vi "Mode Est Process Data.vi"(8 "error in (no error)":errorcluster, 9 "Damping Ratio History":dbl[][](array[numeric]), 10 "Mode Estimator Processing Settings":T3={"Low-Pass Filter Order"=5, "Downsampling Ratio"=10.0, "LPF Cut-off Frequency [Hz]"=2.5, "Sampling Frequency (Hz)"=50.0, "Parcel Length (Simulation)"=30000, "Detrend Cut-off Frequency (Hz)"=0.05, "AR Order"=25, "MA Order "=10, "Lower Frequency [Hz]"=0.08, "Upper Frequency [Hz]"=2.0, "Upper Damping [%]"=20.0, "Lower Damping [%]"=0.0, "Std Threshold"=1.35, "Length of Spectra [s]"=12.0, "Refresh Rate [s]"=0, "Number of critical modes"=1}, 11 "Waveform in":waveform(dbl)) -> (0 "error out":errorcluster, 1 "Display Data B":T2={"Damping ratio evolution"=[], "Estimated Complex Plane"={[], []}, "Critical Frequency [Hz]"=0.0, "Critical Damping [%]"=0.0, " Complex Poles"=[0.0+0.0i, 0.0+0.0i, 0.0+0.0i], "Damping Ratio [%]"=[0.0, 0.0, 0.0], " Frequency[Hz]"=[0.0, 0.0, 0.0], "Mean Damping [%]"=[0.0, 0.0, 0.0], "Pictures"=[bytes[260130], bytes[260130], bytes[260130]], "Std of Damping"=[0.0, 0.0, 0.0]} {"Frequency[Hz]" format="%.4f"; "Damping Ratio [%]" format="%.4f"; "Complex Poles" format="%.4f"}, 3 "Display Data A":T1={"Real-time data"={"t0"=timestamp(3467964116.0127993 s since 1904-01-01), "dt"=0.02, "Y"=array[30000 elements]}, "Preprocessed data"={"t0"=timestamp(3467964116.0127993 s since 1904-01-01), "dt"=0.2, "Y"=array[3000 elements]}, "ARMA Transfer Function"=bytes[0], "Spectrogram"=[refnum], "Spectrum"={"f0"=0.0, "df"=0.0048828125, "S(f)"=[]}, "Parcel Length (SDK or Simulation)"=30000})   [LabVIEW 2017]
uses:
  Mode Est Processing Settings.ctl
  Display Data B.ctl
  Display Data A.ctl
  <vilib>/Math Plots/3D Math Plots/3D Surface/3D Surface Datatype/3D Surface Datatype.lvclass
  <vilib>/Math Plots/3D Math Plots/3D Surface/3D Surface XCtrl/3D Surface.xctl
  Processing State.ctl
  <vilib>/Math Plots/3D Math Plots/3D Plot/3D Plot Datatype/3D Plot Datatype.lvclass
  <vilib>/addons/Wavelet Analysis/application.llb/WA Detrend (Waveform).vi
  Program Files (x86)/National Instruments/LabVIEW 2017/vi.lib/addons/System Identification/Data Preprocess.llb/SI Lowpass Filter (SISO Waveform).vi
  <vilib>/addons/Time Series Analysis/Modeling and Prediction.llb/TSA ARMA Modeling (Waveform).vi
  <vilib>/addons/Control Design/_Model Construction/Model Creation.llb/Model Creation SubVI/cd_Create Transfer Function Model.vi
  <vilib>/addons/Control Design/_Utility/Model Viewer.llb/Model Viewer SubVI/cd_Draw Transfer Function Equation (TF).vi
  <vilib>/addons/Control Design/_Model Conversions/Continuous and Discrete.llb/Continuous and Discrete SubVI/cd_Convert Discrete to Continuous (TF).vi
  <vilib>/addons/Control Design/_Model Conversions/Model Type.llb/Model Conversion SubVI/cd_Convert Transfer Function to State-Space Model.vi
  <vilib>/addons/Control Design/_Dynamic Analysis/Dynamic Analysis.llb/Dynamic Analysis subVI/cd_Damping Ratio and Natural Frequency (State-Space).vi
  <vilib>/imath/engines/lvmath2/RunTimeEngine/Managers/WorkSpace/UID Generator.vi
  <vilib>/imath/engines/lvmath2/RunTimeEngine/BuiltInFunctions/sort/NIMS_[2o]_sort(RRowV,I32,Str).vi
  <instcachedir>/0/NIMS_[2o]_sort(RRowV,I32,Str)_E84E23B068DF4763991B1E74560868DE.lvgen/NIMS_[2o]_sort(RRowV,I32,Str)_E84E23B068DF4763991B1E74560868DE_000.vi
  <vilib>/imathl/engines/lvmath/Functions/Error Handling/Create Error.vi
  <vilib>/imath/engines/lvmath2/RunTimeEngine/IndexRead/NIMS V(V).vi
  <instcachedir>/0/NIMS V(V)_298D9CB7BFEB42B8BC8D9C3C28AE8C70.lvgen/NIMS V(V)_298D9CB7BFEB42B8BC8D9C3C28AE8C70_000.vi
  <instcachedir>/0/NIMS V(V)_298D9CB7BFEB42B8BC8D9C3C28AE8C70.lvgen/NIMS V(V)_298D9CB7BFEB42B8BC8D9C3C28AE8C70_001.vi
  <vilib>/imath/engines/lvmath2/RunTimeEngine/BitwiseOperatorToken/NIMS_Bitwise_Operator_And.vi
  <instcachedir>/0/NIMS_Bitwise_Operator_And_BF79565AECDF4B89921EA9614C6BB008.lvgen/NIMS_Bitwise_Operator_And_BF79565AECDF4B89921EA9614C6BB008_001.vi
  <vilib>/imath/engines/lvmath2/RunTimeEngine/BuiltInFunctions/imag/NIMS_imag(Complex).vi
  <instcachedir>/0/NIMS_imag(Complex)_3180D40D00C843A49C2B33397F857BF3.lvgen/NIMS_imag(Complex)_3180D40D00C843A49C2B33397F857BF3_002.vi
  <vilib>/imath/engines/lvmath2/RunTimeEngine/BuiltInFunctions/findnz/NIMS_[1o]_findnz(GRowV).vi
  <instcachedir>/0/NIMS_[1o]_findnz(GRowV)_4566141FE5BA40B7B10E18ED0AB78B2D.lvgen/NIMS_[1o]_findnz(GRowV)_4566141FE5BA40B7B10E18ED0AB78B2D_000.vi
  <vilib>/imath/engines/lvmath2/RunTimeEngine/RunTimeType/NIMS_RunTimeType_From StrictType (excl LVString).vi
  <instcachedir>/0/NIMS_RunTimeType_From StrictType (excl LVString)_DC56D72BB6B948F98D63F1A957D87C42.lvgen/NIMS_RunTimeType_From StrictType (excl LVString)_DC56D72BB6B948F98D63F1A957D87C42_000.vi
  <vilib>/imath/engines/lvmath2/RunTimeEngine/ErrorHandling/NIMS_Create Error From Enums.vi
  <vilib>/imath/engines/lvmath2/RunTimeEngine/LocalVariableDefStatement/MC_LocalVariableDefStatement_Display.vi
  <vilib>/imath/engines/lvmath2/RunTimeEngine/Managers/SymbolTable/Clear UID.vi
  <vilib>/imath/engines/lvmath2/RunTimeEngine/NodeEndStatement/NIMS_NodeEndStatement_Output.vi
  <instcachedir>/0/NIMS_NodeEndStatement_Output_53EC0D466D134D7ABD903AC30B43404B.lvgen/NIMS_NodeEndStatement_Output_53EC0D466D134D7ABD903AC30B43404B_005.vi
  <instcachedir>/0/NIMS_NodeEndStatement_Output_53EC0D466D134D7ABD903AC30B43404B.lvgen/NIMS_NodeEndStatement_Output_53EC0D466D134D7ABD903AC30B43404B_000.vi
  <vilib>/imath/engines/lvmath2/RunTimeEngine/ErrorHandling/NIMS_Finalize Error.vi
  <vilib>/addons/Time Series Analysis/Correlation and Spectral Analysis.llb/TSA ARMA Spectrum (Waveform).vi
  <vilib>/imath/engines/lvmath2/RunTimeEngine/RangeToken/NIMS_Range.vi
  <instcachedir>/0/NIMS_Range_8C005833F4504FD4A29AA23D6150121A.lvgen/NIMS_Range_8C005833F4504FD4A29AA23D6150121A_000.vi
  <vilib>/imath/engines/lvmath2/RunTimeSupport/NIMS_Error if Not Equal.vi
  <instcachedir>/0/NIMS_Error if Not Equal_E5646C1EFB50404BB0542B8CFB81CE27.lvgen/NIMS_Error if Not Equal_E5646C1EFB50404BB0542B8CFB81CE27_001.vi
  <instcachedir>/0/NIMS_Error if Not Equal_E5646C1EFB50404BB0542B8CFB81CE27.lvgen/NIMS_Error if Not Equal_E5646C1EFB50404BB0542B8CFB81CE27_000.vi
  <vilib>/imath/engines/lvmath2/RunTimeEngine/IndexRead/NIMS V($).vi
  <instcachedir>/0/NIMS V($)_C593F32C7F6B43C7B1793952E292524F.lvgen/NIMS V($)_C593F32C7F6B43C7B1793952E292524F_001.vi
  <vilib>/imath/engines/lvmath2/RunTimeEngine/IndexReplace/NIMS M(S,$)=V.vi
  <instcachedir>/0/NIMS M(S,$)=V_552265ADF67C4F4FB07E91CD22492551.lvgen/NIMS M(S,$)=V_552265ADF67C4F4FB07E91CD22492551_000.vi
  <vilib>/imath/engines/lvmath2/RunTimeEngine/IndexReplace/NIMS V(S)=S.vi
  <instcachedir>/0/NIMS V(S)=S_EDDEB2B900FD4B108B325BCE58B17C3D.lvgen/NIMS V(S)=S_EDDEB2B900FD4B108B325BCE58B17C3D_000.vi
  <vilib>/imath/engines/lvmath2/RunTimeEngine/IndexReplace/NIMS V(V)=V.vi
  <instcachedir>/0/NIMS V(V)=V_ACB9F458E2974419B362D656D10048D7.lvgen/NIMS V(V)=V_ACB9F458E2974419B362D656D10048D7_000.vi
  <vilib>/imath/engines/lvmath2/RunTimeEngine/IndexRead/NIMS M(V,$).vi
  <instcachedir>/0/NIMS M(V,$)_21A5155762F74C04AE4EA67BEE0D3EF5.lvgen/NIMS M(V,$)_21A5155762F74C04AE4EA67BEE0D3EF5_004.vi
  <instcachedir>/0/NIMS_NodeEndStatement_Output_53EC0D466D134D7ABD903AC30B43404B.lvgen/NIMS_NodeEndStatement_Output_53EC0D466D134D7ABD903AC30B43404B_009.vi
  <instcachedir>/0/NIMS_NodeEndStatement_Output_53EC0D466D134D7ABD903AC30B43404B.lvgen/NIMS_NodeEndStatement_Output_53EC0D466D134D7ABD903AC30B43404B_002.vi
  <instcachedir>/0/NIMS_NodeEndStatement_Output_53EC0D466D134D7ABD903AC30B43404B.lvgen/NIMS_NodeEndStatement_Output_53EC0D466D134D7ABD903AC30B43404B_001.vi
  <vilib>/Math Plots/3D Math Plots/3D Surface/3D Surface Datatype/Public/Plot Helper (Vector).vi
  <vilib>/addons/Control Design/_Model Construction/Data Typedefs.llb/CD DtoC Conversion Method.ctl
  Program Files (x86)/National Instruments/LabVIEW 2017/vi.lib/addons/System Identification/NI_SysID.lvlib
  <vilib>/addons/_Advanced Signal Processing/NI_AdvSigProcWA.lvlib
  <vilib>/addons/_Advanced Signal Processing/NI_AdvSigProcTSA.lvlib
  <vilib>/addons/Control Design/_Model Construction/NI_LinSys_Model Creation.lvlib
  <vilib>/addons/Control Design/_Model Conversions/NI_CD_Continuous and Discrete.lvlib
  <vilib>/addons/Control Design/_Model Construction/NI_LinSys_Data Typedefs.lvlib
  <vilib>/addons/Control Design/_Dynamic Analysis/NI_CD_Dynamic Analysis.lvlib
  <vilib>/Analysis/NI_AALBase.lvlib
  <vilib>/addons/Control Design/_Model Conversions/NI_CD_Model Type.lvlib
  <vilib>/imath/engines/lvmath2/RunTimeEngine/Managers/SymbolTable/NIMS_WorkSpace.lvlib
  <vilib>/addons/Control Design/_Utility/NI_CD_Model Viewer.lvlib
panel:
  # "MA\n_______\n\n   AR"
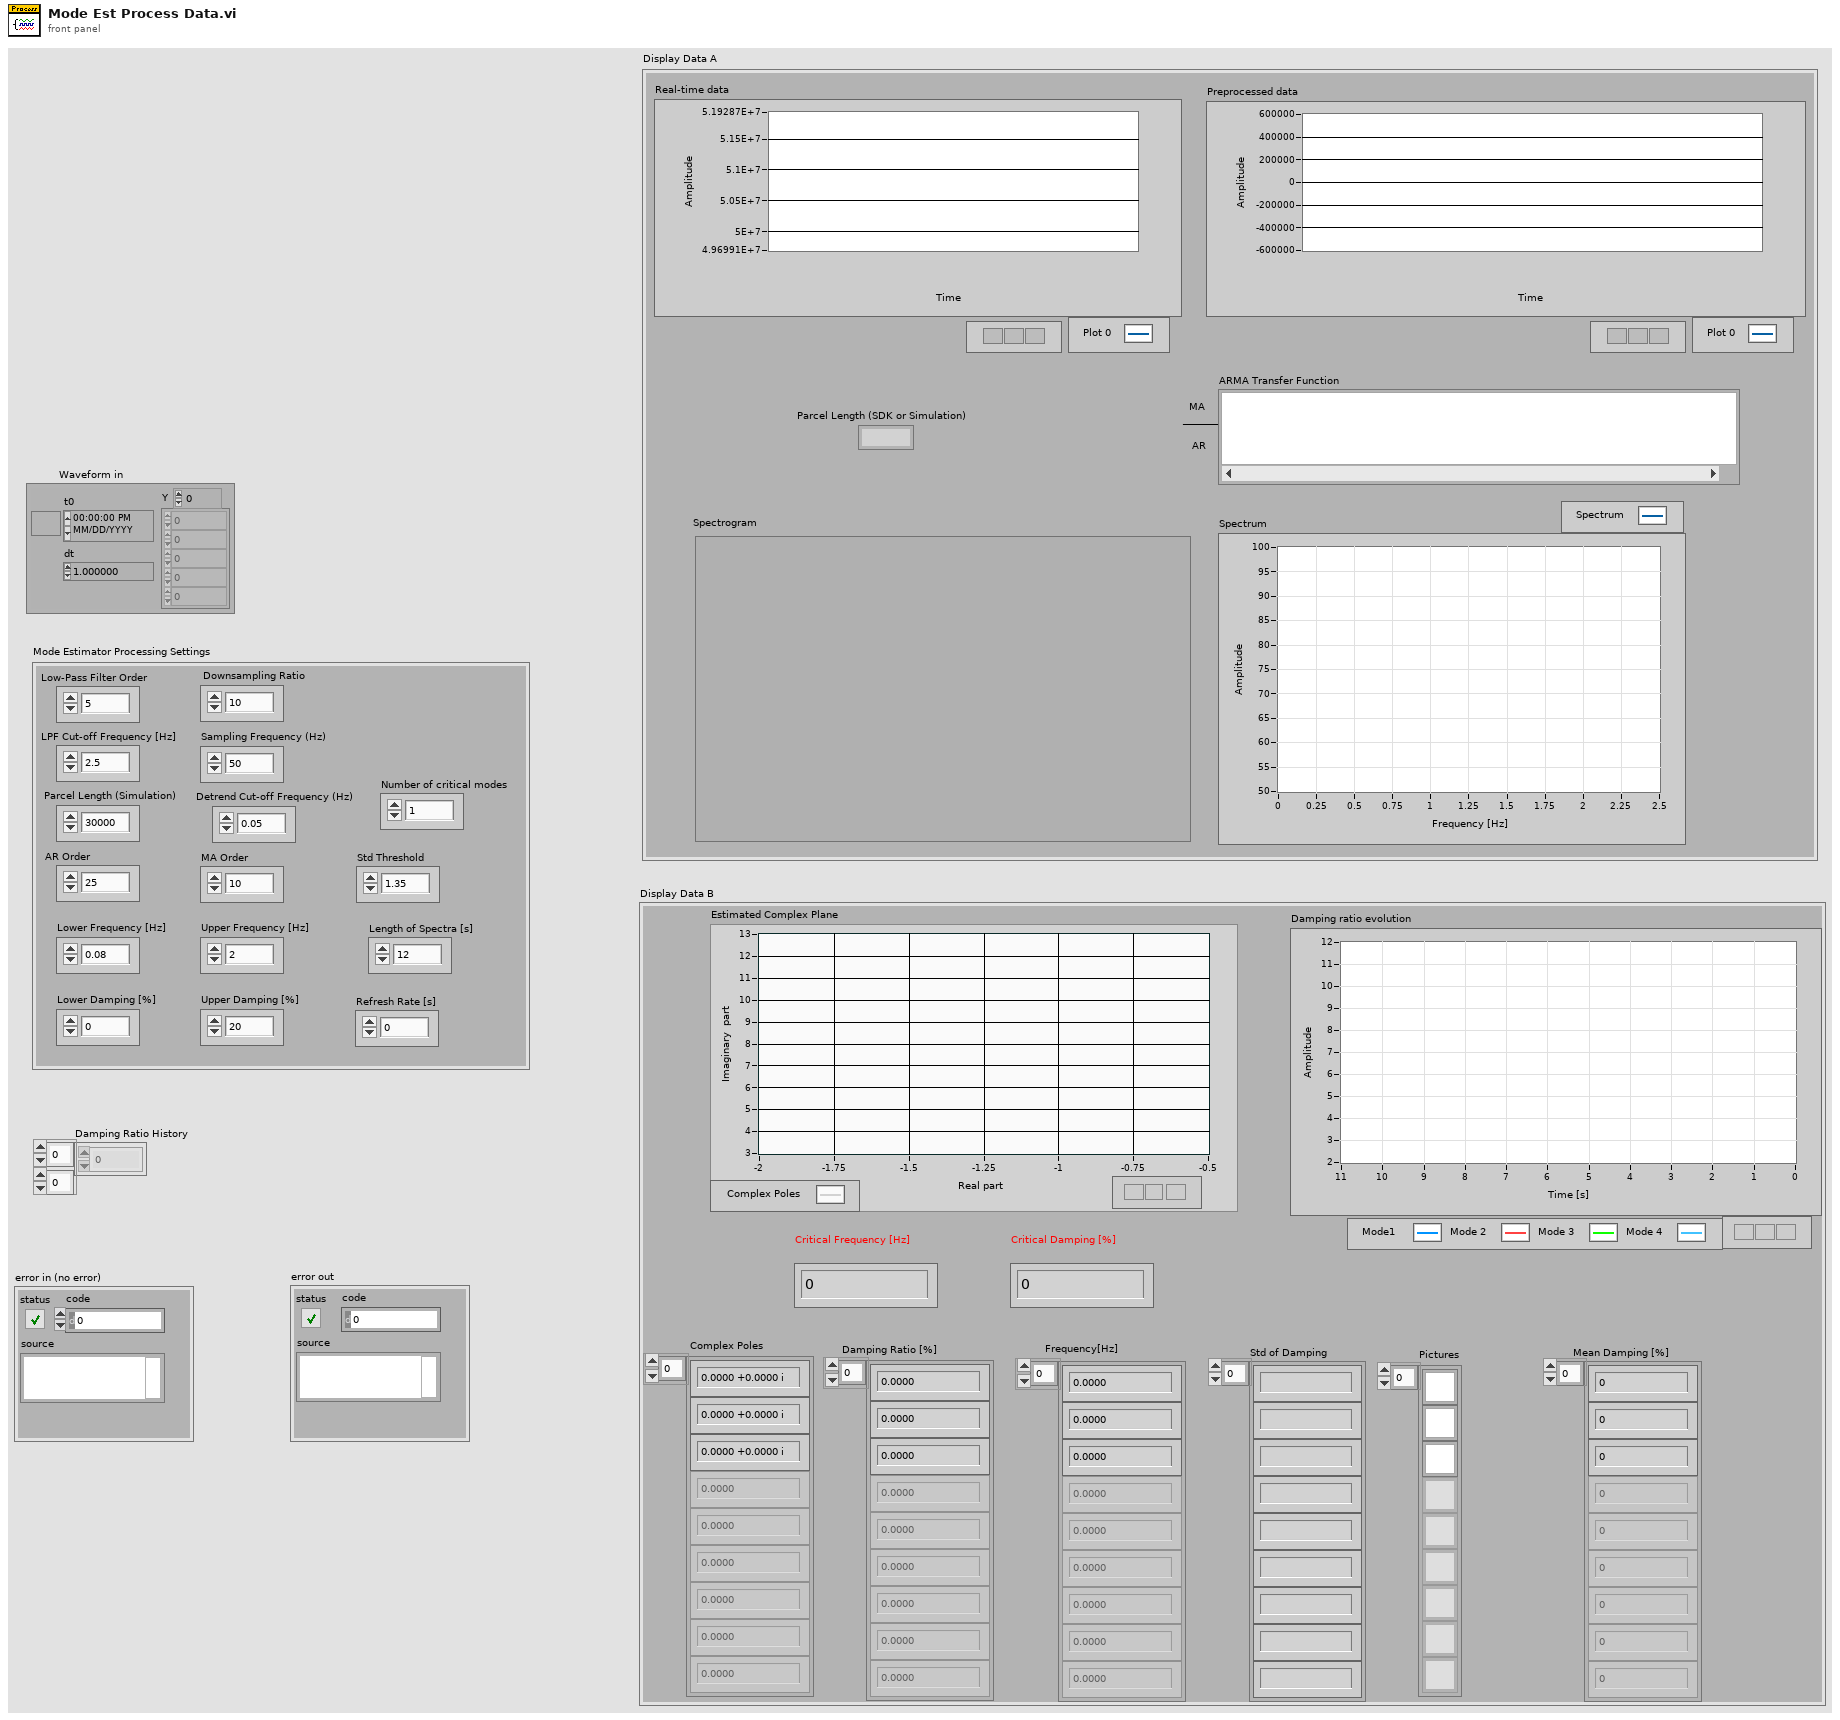
[diagram p1: front panel]
types:
  T1 = typedef "Display Data A.ctl" = cluster{"Real-time data":waveform(dbl), "Preprocessed data":waveform(dbl), "ARMA Transfer Function":picture, "Spectrogram":refnum<class "3D Plot Datatype.lvclass">[], "Spectrum":cluster{"f0":dbl, "df":dbl, "S(f)":dbl[]}, "Parcel Length (SDK or Simulation)":i32}
  T2 = typedef "Display Data B.ctl" = cluster{"Damping ratio evolution":dbl[][], "Estimated Complex Plane":cluster{dbl[], dbl[]}, "Critical Frequency [Hz]":dbl, "Critical Damping [%]":dbl, " Complex Poles":cdb[], "Damping Ratio [%]":dbl[], " Frequency[Hz]":dbl[], "Mean Damping [%]":dbl[], "Pictures":picture[], "Std of Damping":dbl[]}
  T3 = typedef "Mode Est Processing Settings.ctl" = cluster{"Low-Pass Filter Order":i32, "Downsampling Ratio":dbl, "LPF Cut-off Frequency [Hz]":dbl, "Sampling Frequency (Hz)":dbl, "Parcel Length (Simulation)":i32, "Detrend Cut-off Frequency (Hz)":dbl, "AR Order":i32, "MA Order ":i32, "Lower Frequency [Hz]":dbl, "Upper Frequency [Hz]":dbl, "Upper Damping [%]":dbl, "Lower Damping [%]":dbl, "Std Threshold":dbl, "Length of Spectra [s]":dbl, "Refresh Rate [s]":i32, "Number of critical modes":i32}
  T4 = typedef "Processing State.ctl" = enum16{"Preprocessing", "Compute AR Coeff", "Get Spectrum"}
  T5 = cluster{"Damping ratio evolution":dbl[][], "Estimated Complex Plane":cluster{dbl[], dbl[]}, "Critical Frequency [Hz]":dbl, "Critical Damping [%]":dbl, " Complex Poles":cdb[], "Damping Ratio [%]":dbl[], " Frequency[Hz]":dbl[], "Mean Damping [%]":dbl[], "Pictures":picture[], "Std of Damping":dbl[]}
  T6 = typedef "NI_LinSys_Data Typedefs.lvlib/CD DtoC Conversion Method.ctl" = u16
  T7 = typedef "NI_LinSys_Model Typedefs.lvlib/CD Transfer Function Model (MIMO).ctl" = cluster{"properties":T8, "transfer function(s)":T9[][]}
  T8 = typedef "NI_LinSys_Model Typedefs.lvlib/CD General Elements.ctl" = cluster{"Model name":string, "Input names":string[], "Output names":string[], "Input Delays":dbl[], "Output Delays":dbl[], "Sampling Time":dbl, "Notes":string}
  T9 = typedef "NI_LinSys_Model Typedefs.lvlib/CD Transfer Function Model (SISO).ctl" = cluster{"Numerator":dbl[], "Denominator":dbl[], "delay":dbl}
  T10 = typedef "NI_LinSys_Model Typedefs.lvlib/CD State Space Model (MIMO).ctl" = cluster{"properties":T8, "A":dbl[][], "B":dbl[][], "C":dbl[][], "D":dbl[][], "StateNames":string[], "Transport Delay":dbl[][]}
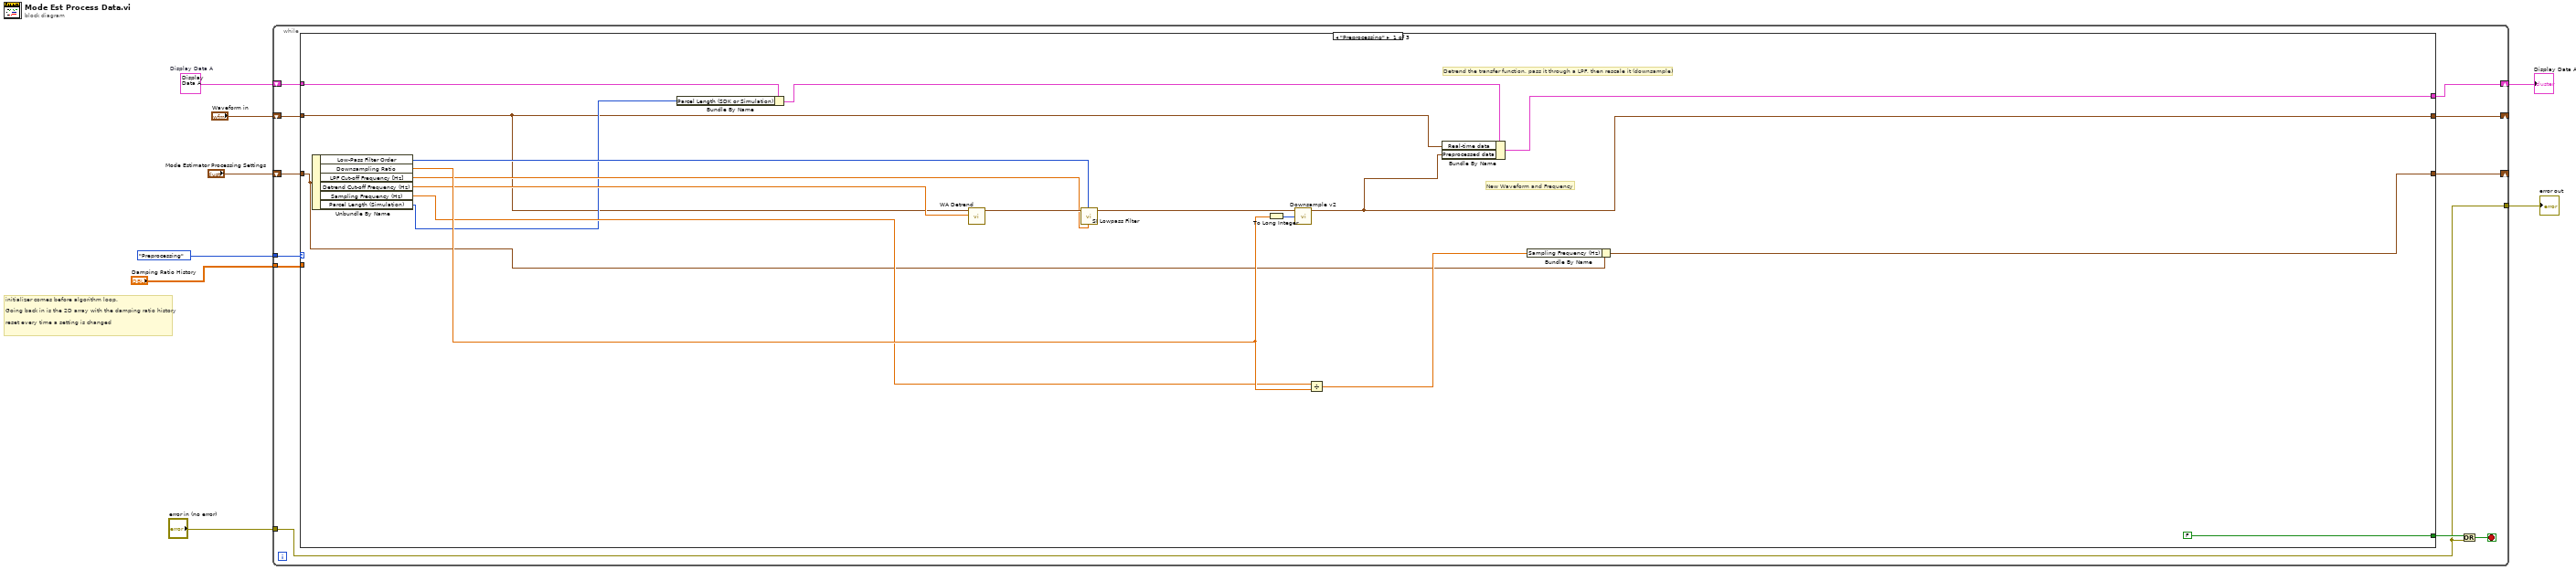
[diagram p0: block diagram]
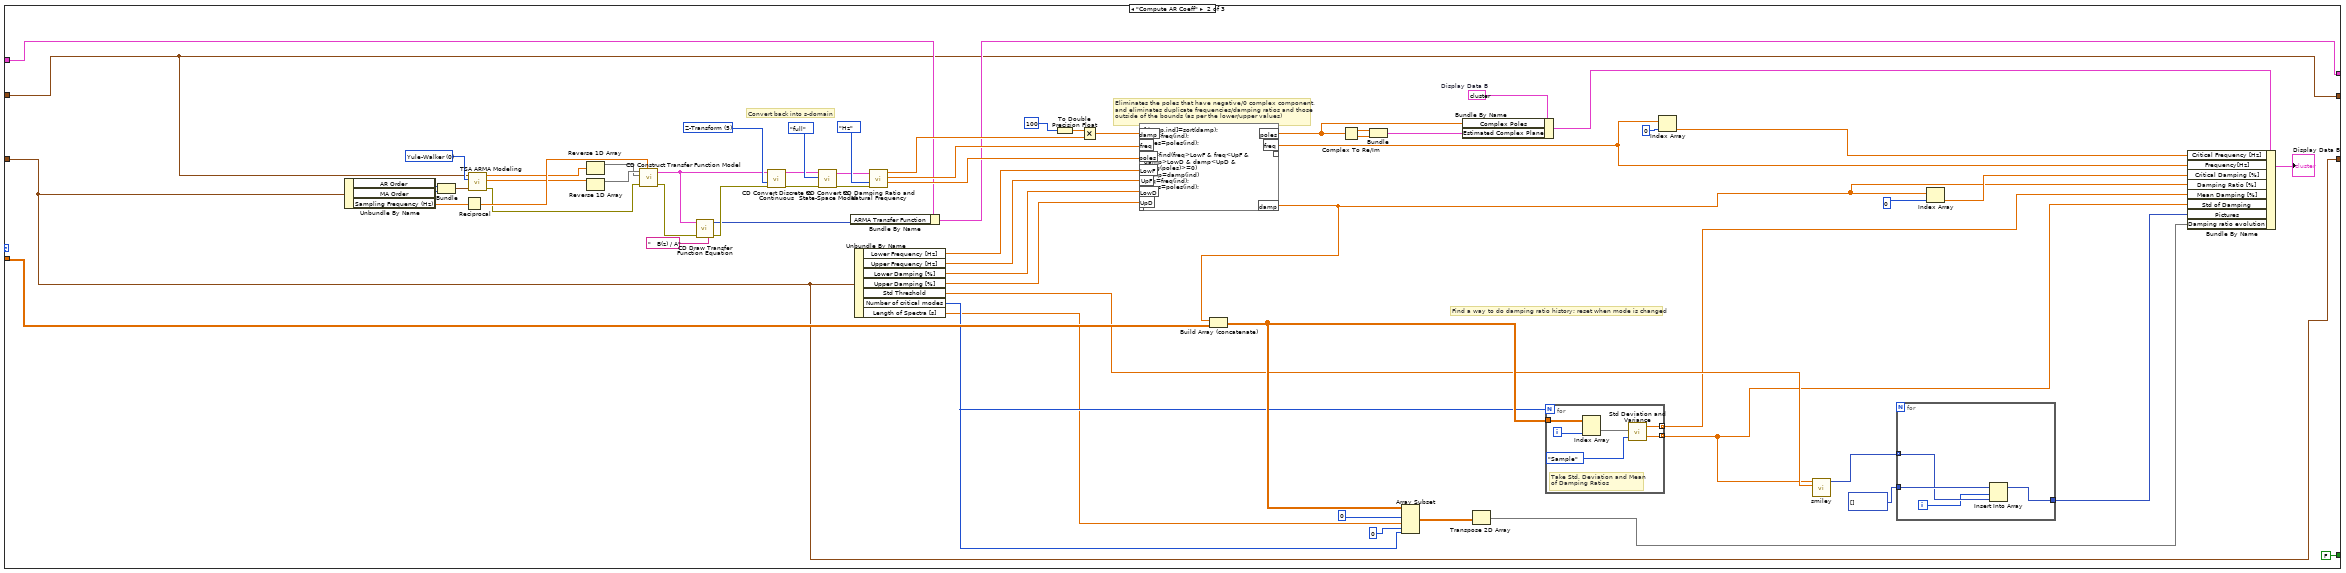
[diagram p2: hidden frame]
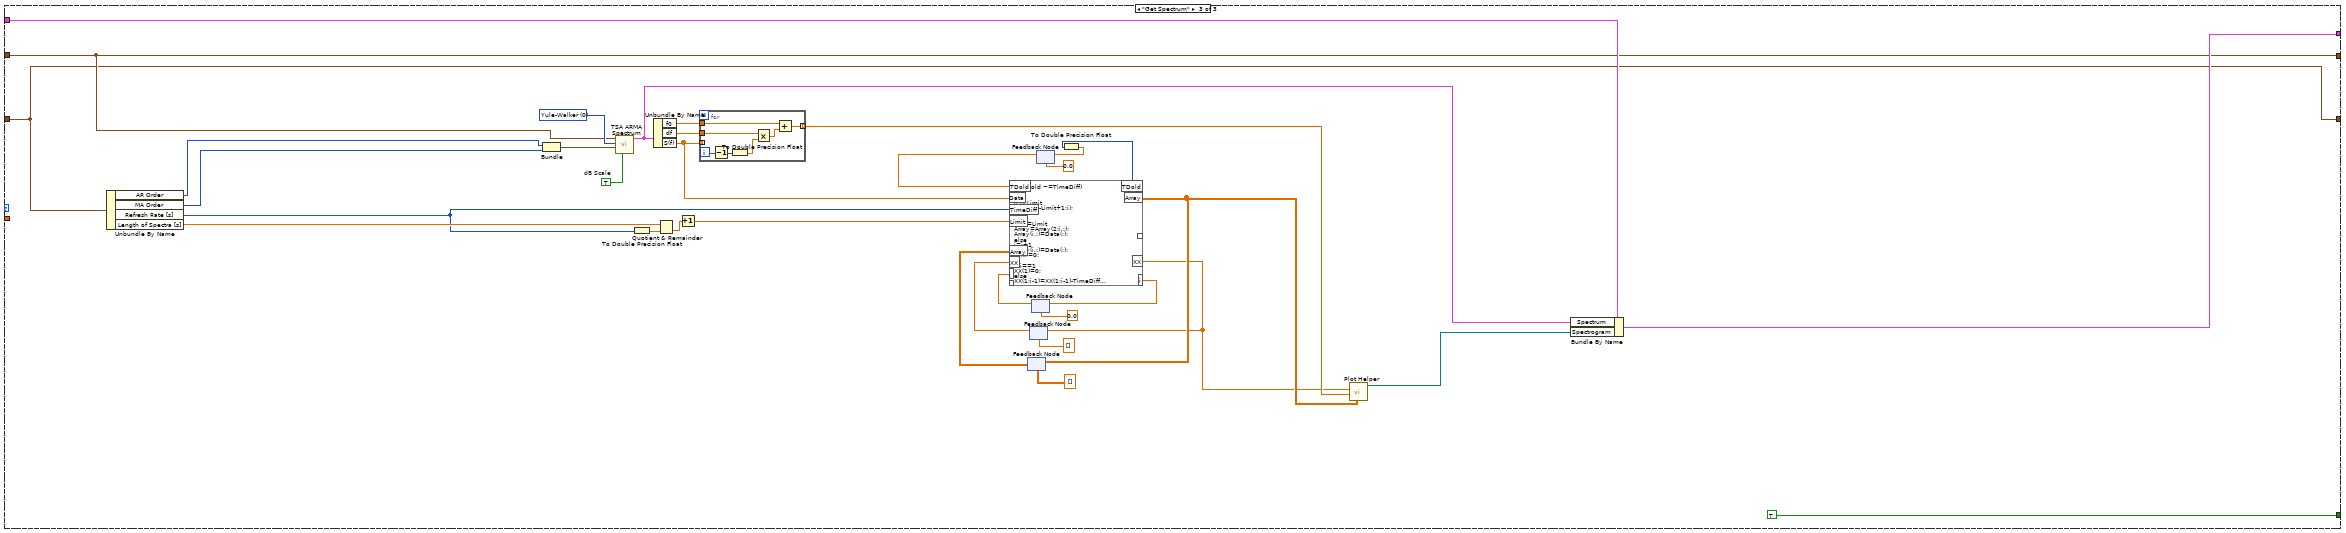
[diagram p3: hidden frame]
diagram:
  w4 = T1 {"Real-time data"={"t0"=timestamp(3467964116.0127993 s since 1904-01-01), "dt"=0.02, "Y"=array[30000 elements]}, "Preprocessed data"={"t0"=timestamp(3467964116.0127993 s since 1904-01-01), "dt"=0.2, "Y"=array[3000 elements]}, "ARMA Transfer Function"=bytes[0], "Spectrogram"=[refnum], "Spectrum"={"f0"=0.0, "df"=0.0048828125, "S(f)"=[]}, "Parcel Length (SDK or Simulation)"=30000}  # Display Data A
  # "initializer comes before algorithm loop.\n\nGoing back in is the 2D array with the damping ratio history\n\nreset every time a setting is changed"
  n1 = while {
    tunnel: "Damping Ratio History" -> [w19]
    tunnel: Processing_State."Preprocessing" ("Enum") -> [w17]
    shift-right: [w16] -> _
    shift-left: "Waveform in" -> [w10]
    shift-right: [w15] -> w5
    shift-left: w4 -> [w14]
    tunnel: "error in (no error)" -> [w11]
    tunnel: [w11] -> w2
    shift-right: [w9] -> _
    shift-left: "Mode Estimator Processing Settings" -> [w18]
    stop <- w12 stop-if-true
    n2 = case shown="\"Preprocessing\"" w17 {
      tunnel: w10 -> [w26 w39 w330]
      tunnel: [w21 w39 w330] -> w16
      tunnel: w19 -> [_ w96 _]
      tunnel: w18 -> [w23 w38 w329]
      tunnel: [FALSE FALSE TRUE] -> w13
      tunnel: w14 -> [w30 w41 w334]
      tunnel: [w31 w40 w333] -> w15
      tunnel: [w24 w38 w329] -> w9
      frame "Preprocessing" {
        # "New Waveform and Frequency"
        # "Detrend the transfer function, pass it through a LPF, then rescale it (downsample)"
        n3 = Unbundle By Name(w23) -> ("Low-Pass Filter Order"=w36:i32, "Downsampling Ratio"=w35:dbl, "LPF Cut-off Frequency [Hz]"=w34:dbl, "Detrend Cut-off Frequency (Hz)"=w33:dbl, "Sampling Frequency (Hz)"=w28:dbl, "Parcel Length (Simulation)"=w27:i32)
        n4 = Bundle By Name(cluster=w30, "Parcel Length (SDK or Simulation)"=w27) -> (w29:T1)
        n5 = call-poly <vilib>:"WA Detrend.vi"("threshold frequency"=w33, "signal"=w26) -> ("detrended signal"=w37:waveform(dbl))  [unwired: 7 in, 2 out]
        n6 = call-poly "SI Lowpass Filter.vi"("cutoff frequency"=w34, "order"=w36, "stimulus signal in"=w37) -> ("stimulus signal out"=w22:waveform(dbl))  [unwired: 6 in, 2 out]
        n7 = To Long Integer(number=w35) -> (32bit integer=w20:i32)
        n8 = call "Downsample v2.vi"("Divide by"=w20, "Waveform in"=w22) -> ("Waveform out"=w21:waveform(dbl))  [unwired: 9 in]
        n9 = Divide(x=w28, y=w35) -> (x/y=w25:dbl)
        n10 = Bundle By Name(cluster=w29, "Real-time data"=w26, "Preprocessed data"=w21) -> (w31:T1)
        n11 = Bundle By Name(cluster=w23, "Sampling Frequency (Hz)"=w25) -> (w24:T3)
      }
      frame "Compute AR Coeff" {
        w45 = T5 {"Damping ratio evolution"=[], "Estimated Complex Plane"={[], []}, "Critical Frequency [Hz]"=0.0, "Critical Damping [%]"=0.0, " Complex Poles"=[0.0+0.0i, 0.0+0.0i, 0.0+0.0i], "Damping Ratio [%]"=[0.0, 0.0, 0.0], " Frequency[Hz]"=[0.0, 0.0, 0.0], "Mean Damping [%]"=[0.0, 0.0, 0.0], "Pictures"=[bytes[260130], bytes[260130], bytes[260130]], "Std of Damping"=[0.0, 0.0, 0.0]}  # Display Data B
        w101 = T6 5 items=["Zero-Order-Hold", "Tustin (Bilinear)", "Prewarp", "Forward", "Backward", "Z-Transform"] ("Method")
        w102 = u16 0 items=["Yule-Walker", "High order AR", "Polynomial"] ("method")
        # "Find a way to do damping ratio history; reset when mode is changed"
        # "Convert back into s-domain"
        # "Eliminates the poles that have negative/0 complex component,\nand eliminates duplicate frequencies/damping ratios and those \noutside of the bounds (as per the lower/upper values)"
        n12 = Unbundle By Name(w38) -> ("AR Order"=w100:i32, "MA Order"=w76:i32, "Sampling Frequency (Hz)"=w74:dbl)
        n13 = Bundle("AR Order"=w100, "MA Order"=w76) -> (w99:cluster{"AR Order":i32, "MA Order ":i32})  [unwired: 1 in]
        n14 = Reciprocal(x=w74) -> (1/x=w75:dbl)
        n15 = call-poly <vilib>:"TSA ARMA Modeling.vi"("ARMA order"=w99, "method"=w102, "Xt"=w39) -> ("error out"=w66:errorcluster, "MA coefficients"=w71:dbl[], "AR coefficients"=w72:dbl[])  [unwired: 5 in, 1 out]
        n16 = Reverse 1D Array(array=w72) -> (reversed array=w88:dbl[])
        n17 = Reverse 1D Array(array=w71) -> (reversed array=w89:dbl[])
        n18 = call-poly <vilib>:"CD Construct Transfer Function Model.vi"("Sampling Time (s)"=w75, "error in (no error)"=w66, "Denominator"=w88, "Numerator"=w89) -> ("error out"=w68:errorcluster, "Transfer Function Model"=w70:T7)  [unwired: 6 in]
        n19 = call-poly <vilib>:"CD Draw Transfer Function Equation.vi"("Function Name (empty)"="   B(z) / A", "error in (no error)"=w68, "Transfer Function Model"=w70) -> ("error out"=w67:errorcluster, "Equation"=w42:picture)  [unwired: 6 in, 1 out]
        n20 = call-poly <vilib>:"CD Convert Discrete to Continuous.vi"("error in (no error)"=w67, "Method"=w101, "Discrete Transfer Function Model"=w70) -> ("error out"=w83:errorcluster, "Continuous Transfer Function Model"=w80:T7)  [unwired: 7 in]
        n21 = call-poly <vilib>:"CD Convert to State-Space Model.vi"("error in (no error)"=w83, "Realization Type"=enum16{"minimum", "full"}."full", "Transfer Function Model"=w80) -> ("error out"=w79:errorcluster, "State-Space Model"=w81:T10)  [unwired: 7 in]
        n22 = Bundle By Name(cluster=w41, "ARMA Transfer Function"=w42) -> (w40:T1)
        n23 = Unbundle By Name(w38) -> ("Lower Frequency [Hz]"=w62:dbl, "Upper Frequency [Hz]"=w63:dbl, "Lower Damping [%]"=w64:dbl, "Upper Damping [%]"=w65:dbl, "Std Threshold"=w59:dbl, "Number of critical modes"=w58:i32, "Length of Spectra [s]"=w57:dbl)
        n24 = call-poly <vilib>:"CD Damping Ratio and Natural Frequency.vi"("error in (no error)"=w79, "Frequency Unit"=enum16{"Hz", "rad/s"}."Hz", "State-Space Model"=w81) -> ("Poles"=w90:cdb[], "Natural Frequencies"=w84:dbl[], "Damping Ratios"=w93:dbl[])  [unwired: 5 in, 1 out]
        n25 = To Double Precision Float(number=100 ("Numeric")) -> (double precision float=w78:dbl)
        n26 = Multiply(x=w78, y=w93) -> (x*y=w92:dbl[])
        n27 = mathscript code="[damp,ind]=sort(damp);\nfreq=freq(ind);\npoles=poles(ind);\n\nind=find(freq>LowF & freq<UpF & damp>LowD & damp<UpD &  imag(poles)>=0)\ndamp=damp(ind)\nfreq=freq(ind);\npoles=poles(ind);"("damp"=w92, "freq"=w84, "poles"=w90, "LowF"=w62, "UpF"=w63, "LowD"=w64, "UpD"=w65) -> ("poles"=w52:cdb[], "freq"=w50:dbl[], "damp"=w49:dbl[])  [unwired: 1 in, 1 out]
        n28 = Build Array (concatenate) "Build Array"(w49, w96) -> (w61:dbl[][])
        n29 = Complex To Re/Im(x + iy=w52) -> (x=w98:dbl[], y=w97:dbl[])
        n30 = Bundle(w98, w97) -> (w56:cluster{dbl[], dbl[]})  [unwired: 1 in]
        n31 = Array Subset "Array Subset"(array=w61, index (row)=0 ("index"), length (row)=w57, index (col)=0 ("index"), length (col)=w58) -> (w73:dbl[][])
        n32 = Bundle By Name(cluster=w45, "Complex Poles"=w52, "Estimated Complex Plane"=w56) -> (w54:T5)
        n33 = Transpose 2D Array(2D array=w73) -> (transposed array=w48:dbl[][])
        n34 = for {
          N: w58 -> [_]
          tunnel: w61 -> [w111]
          tunnel: [w109] -> w47 mode=indexing
          tunnel: [w108] -> w43 mode=indexing
          i -> [w107]
          # "Take Std. Deviation and Mean\nof Damping Ratios"
          n35 = Index Array "Index Array"(array=w111, index (col)=w107) -> (element=w110:dbl[])  [unwired: 1 in]
          n36 = call <vilib>:"Std Deviation and Variance.vi"("X"=w110, "Weighting (Sample)"=enum16{"Sample", "Population"}."Sample") -> ("mean"=w109:dbl, "standard deviation"=w108:dbl)  [unwired: 1 out]
        }
        n37 = Index Array(array=w50, index=0) -> (element=w55:dbl)
        n38 = call "smiley.vi"("std threshold"=w59, "damp"=w43) -> ("Array"=w91:picture[])  [unwired: 9 in]
        n39 = for {
          tunnel: w91 -> [w105] mode=indexing
          tunnel: picture[] [] -> [w106]
          tunnel: [w103] -> w44
          i -> [w104]
          n40 = Insert Into Array(array=w106, index=w104, new element=w105) -> (w103:picture[])
        }
        n41 = Index Array(array=w49, index=0 ("length")) -> (element=w51:dbl)
        n42 = Bundle By Name(cluster=w54, "Critical Frequency [Hz]"=w55, "Frequency[Hz]"=w50, "Critical Damping [%]"=w51, "Damping Ratio [%]"=w49, "Mean Damping [%]"=w47, "Std of Damping"=w43, "Pictures"=w44, "Damping ratio evolution"=w48) -> (→"Display Data B":T5)
      }
      frame "Get Spectrum" {
        w355 = TRUE  # dB Scale
        w352 = u16 0 items=["Yule-Walker", "High order AR", "Polynomial"] ("method")
        n43 = Unbundle By Name(w329) -> ("AR Order"=w332:i32, "MA Order"=w331:i32, "Refresh Rate [s]"=w337:i32, "Length of Spectra [s]"=w338:dbl)
        n44 = Bundle("AR Order"=w332, "MA Order"=w331) -> (w362:cluster{"AR Order":i32, "MA Order ":i32})  [unwired: 1 in]
        n45 = call-poly <vilib>:"TSA ARMA Spectrum.vi"("dB on? (T)"=w355, "ARMA order"=w362, "method"=w352, "Xt"=w330) -> ("PSD"=w336:cluster{"f0":dbl, "df":dbl, "S(f)":dbl[]})  [unwired: 5 in, 2 out]
        n46 = To Double Precision Float(number=w337) -> (double precision float=w344:dbl)
        n47 = Unbundle By Name(w336) -> ("f0"=w360:dbl, "df"=w359:dbl, "S(f)"=w356:dbl[])
        n48 = Quotient & Remainder(x=w338, y=w344) -> (floor(x/y)=w346:dbl)  [unwired: 1 out]
        n49 = Increment(x=w346) -> (x+1=w345:dbl)
        n50 = for {
          tunnel: w356 -> [_] mode=indexing
          tunnel: w360 -> [w366]
          tunnel: w359 -> [w368]
          tunnel: [w365] -> w351 mode=indexing
          i -> [w369]
          n51 = Decrement(x=w369) -> (x-1=w363:i32)
          n52 = To Double Precision Float(number=w363) -> (double precision float=w364:dbl)
          n53 = Multiply(x=w368, y=w364) -> (x*y=w367:dbl)
          n54 = Add(x=w366, y=w367) -> (x+y=w365:dbl)
        }
        n55 = feedback #1(dbl[][] [] ("Array")) -> (w354:dbl[][])
        n56 = feedback #2(dbl[] [] ("XX")) -> (w358:dbl[])
        n57 = feedback #3(0.0 ("i")) -> (w361:dbl)
        n58 = feedback #4(0.0 ("TDold")) -> (w348:dbl)
        n59 = mathscript code="if (TDold ~=TimeDiff)\ni=0\nend\nif i>Limit\nXX=XX(i-Limit+1:i);\ni=Limit;\nend\nif i==Limit\nArray=Array(2:i,:);\nArray(i,:)=Data(:);\nelse\ni=i+1\nArray(i,:)=Data(:);\nXX(i)=0;\n\nif i==1\nXX(1)=0;\nelse\nXX(1:i-1)=XX(1:i-1)-TimeDiff\nXX(i)=0\nend\nend\n\nTDold=TimeDiff;"("Data"=w356, "Array"=w354, "i"=w361, "Limit"=w345, "XX"=w358, "TimeDiff"=w337, "TDold"=w348) -> ("Array"=w350:dbl[][], "i"=w343:dbl, "XX"=w349:dbl[], "TDold"=w340:i32)  [unwired: 1 in, 1 out]
        n60 = feedback-in #1(w350) -> ()
        n61 = feedback-in #2(w349) -> ()
        n62 = feedback-in #3(w343) -> ()
        n63 = To Double Precision Float(number=w340) -> (double precision float=w341:dbl)
        n64 = feedback-in #4(w341) -> ()
        n65 = call-poly <vilib>:"Plot Helper.vi"("z matrix"=w350, "y vector"=w351, "x vector"=w349) -> ("3D Plot lvclass Array out"=w335:refnum<class "3D Plot Datatype.lvclass">[])  [unwired: 3 in, 5 out]
        n66 = Bundle By Name(cluster=w334, "Spectrum"=w336, "Spectrogram"=w335) -> (w333:T1)
      }
    }
    n67 = Or(x=w13, y=w11) -> (x .or. y?=w12:bool)
  }
  "Display Data A" <- w5
  "error out" <- w2
